vi "Sets and Query the Questionable Data Enable Register.vi"(5 "Enable to Query":bool=TRUE, 7 "Enable to Sets":bool=TRUE, 8 "error in":errorcluster, 10 "Questionable Data Enable Register":u16, 11 "VISA resource name":refnum<visa-resource-name>) -> (0 "error out":errorcluster, 2 "Returns the Questionable Data Enable Register":string, 3 "VISA resource name out":refnum<visa-resource-name>)   [LabVIEW 2011, in "DMM4.lvlib"]
uses:
  <instrlib>/DMM4/DMM4.lvlib
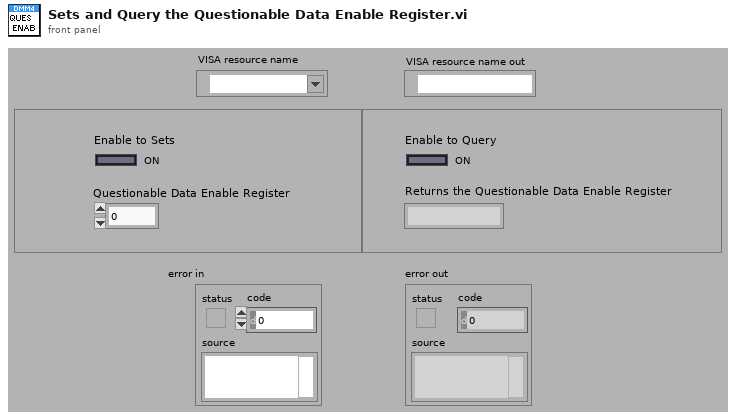
[diagram p1: front panel]
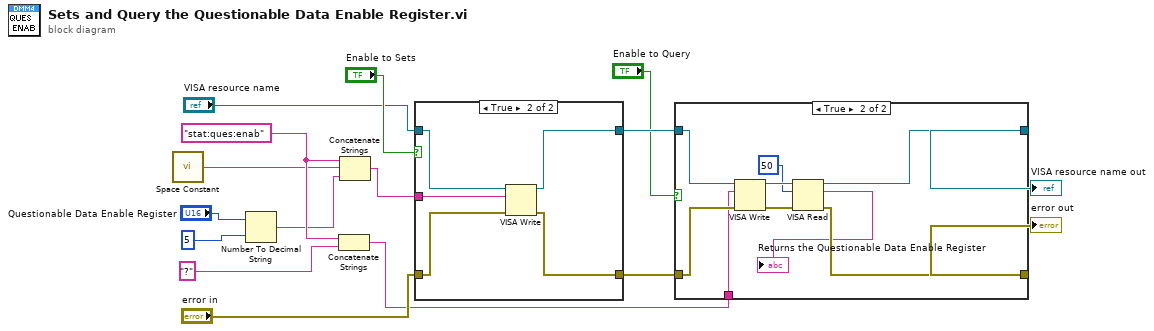
[diagram p0: block diagram]
diagram:
  w5 = "stat:ques:enab"
  n1 = call <vilib>:"Space Constant.vi"() -> ("String"=w4:string)
  n2 = Number To Decimal String(number="Questionable Data Enable Register", width (-)=i16 5) -> (decimal integer string=w3:string)
  n3 = Concatenate Strings(w5, "?") -> (w10:string)
  n4 = Concatenate Strings(w5, w4, w3) -> (w1:string)
  n5 = case shown="True" "Enable to Sets" {
    tunnel: "VISA resource name" -> [w18 w23]
    tunnel: "error in" -> [w17 w22]
    tunnel: [w18 w21] -> w12
    tunnel: [w17 w20] -> w11
    tunnel: w1 -> [_ w19]
    frame False {
    }
    frame True {
      n6 = VISA Write(VISA resource name=w23, write buffer=w19, error in (no error)=w22) -> (VISA resource name out=w21:refnum<visa-resource-name>, error out=w20:errorcluster)  [unwired: 1 out]
    }
  }
  n7 = case shown="True" "Enable to Query" {
    tunnel: w12 -> [w25 w32]
    tunnel: [w25 w30] -> w8
    tunnel: w11 -> [w24 w31]
    tunnel: [w24 w29] -> w7
    tunnel: w10 -> [_ w27]
    frame False {
    }
    frame True {
      n8 = VISA Write(VISA resource name=w32, write buffer=w27, error in (no error)=w31) -> (VISA resource name out=w33:refnum<visa-resource-name>, error out=w34:errorcluster)  [unwired: 1 out]
      n9 = VISA Read(VISA resource name=w33, byte count=u32 50, error in (no error)=w34) -> (VISA resource name out=w30:refnum<visa-resource-name>, read buffer=→"Returns the Questionable Data Enable Register":string, error out=w29:errorcluster)  [unwired: 1 out]
    }
  }
  "VISA resource name out" <- w8
  "error out" <- w7
